vi "Build Runtime Menu.vi"(4 "error in (no error)":errorcluster, 7 "Menu in":refnum<k9>) -> (0 "error out":errorcluster, 3 "Menu out":refnum<k9>)   [LabVIEW 2014, in "Startup Processes.lvlib"]
uses:
  Startup Processes.lvlib
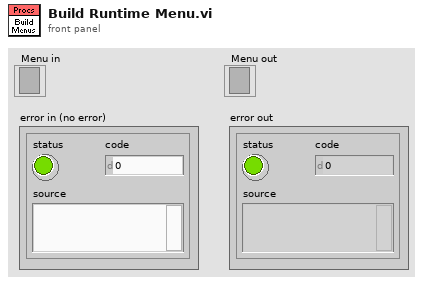
[diagram p1: front panel]
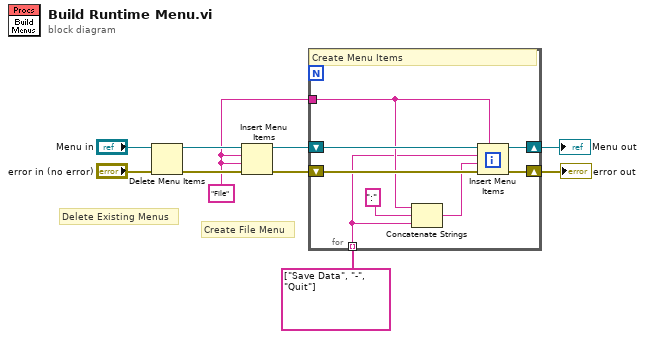
[diagram p0: block diagram]
diagram:
  w2 = "File"
  # "Create File Menu"
  # "Delete Existing Menus"
  n1 = Delete Menu Items(6:"error in (no error)", 9:"Menu in") -> (0:w7:errorcluster, 3:w8:refnum<k9>)  [unwired: 2 in]
  n2 = Insert Menu Items(6:w7, 7:w2, 8:w2, 9:w8) -> (0:w6:errorcluster, 3:w5:refnum<k9>)  [unwired: 2 in, 1 out]
  n3 = for {
    shift-right: [w17] -> w3
    shift-left: w5 -> [w16]
    shift-right: [w18] -> w4
    shift-left: w6 -> [w15]
    tunnel: w2 -> [w12]
    tunnel: string[] ["Save Data", "-", "Quit"] -> [w11] mode=indexing
    # "Create Menu Items"
    n4 = Concatenate Strings(w12, ":" ("string"), w11) -> (w13:string)
    n5 = Insert Menu Items(5:w12, 6:w15, 7:w13, 8:w11, 9:w16) -> (0:w18:errorcluster, 3:w17:refnum<k9>)  [unwired: 1 in, 1 out]
  }
  "Menu out" <- w3
  "error out" <- w4
